vi "6. References.vi"() -> ()   [LabVIEW 2017]
uses:
  6276dcbc-c98b-42be-a14e-8777d527878b.vi
  f718c417-406b-4765-8f4e-f4eec60edb5e.vi
  6276dcbc-c98b-42be-a14e-8777d527878b.vi/b09b9099-6be0-413b-8afc-4908471460c3.vi
  f718c417-406b-4765-8f4e-f4eec60edb5e.vi/b09b9099-6be0-413b-8afc-4908471460c3.vi
  INI-Static-Variable-Support/_Support/global-csm-ini-db-change-flag.vi
  <vilib>/Utility/Data Type/Get Type Information.vi
  <userlib>/_NEVSTOP/Communicable State Machine(CSM)/addons/API-String-Arugments-Support/_Support/Data To SingleElementsArray_csm.vi
  INI-Static-Variable-Support/_Support/Parse Used Session and Name.vi
  <userlib>/_NEVSTOP/Communicable State Machine(CSM)/addons/API-String-Arugments-Support/_Support/Data To API String Arguments.vi
  INI-Static-Variable-Support/_Support/INI-FGV.vi
  <userlib>/_NEVSTOP/Communicable State Machine(CSM)/addons/API-String-Arugments-Support/_Support/Convert API String Arguments to Data(variant).vi
  <userlib>/_NEVSTOP/Communicable State Machine(CSM)/addons/API-String-Arugments-Support/_Support/SingleElementsArray To Data_csm.vi
  INI-Static-Variable-Support/INI-Static-Variable-Support.lvlib
panel:
  out "${NETWORK.URL}":string
  out "${RT.ADDR}":string
  out "case1.addr":string
  out "case2.addr":string
  out "config out 2":cluster{"select":string, "addr":string}
  out "${rt.addr}":string
  out "${network.url} 2":string
  out "${network.url}":string
  out "config out":cluster{"url":string, "host":string}
  out "url":string
  out "host":string
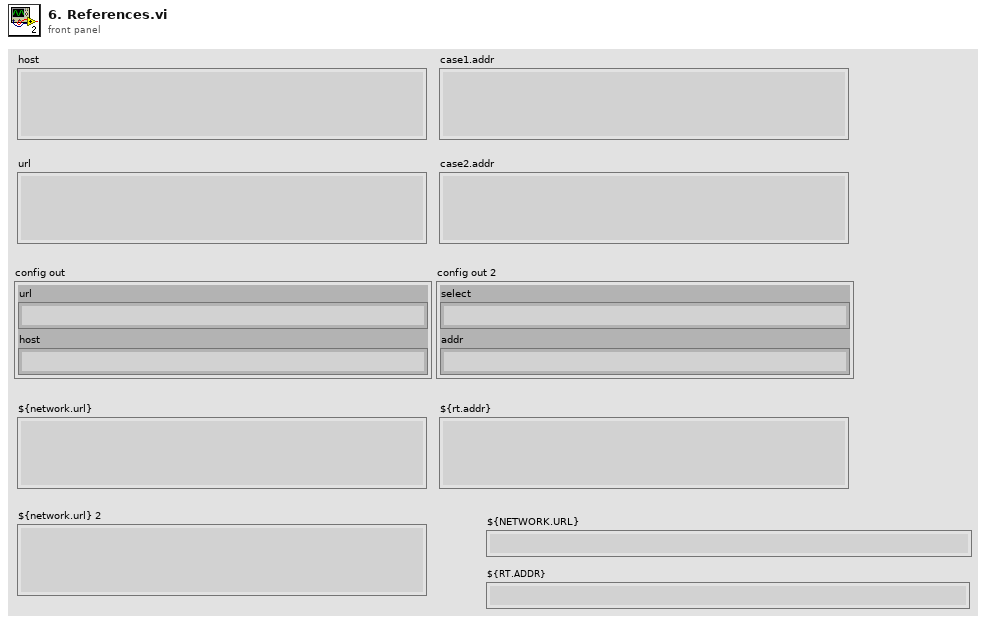
[diagram p1: front panel]
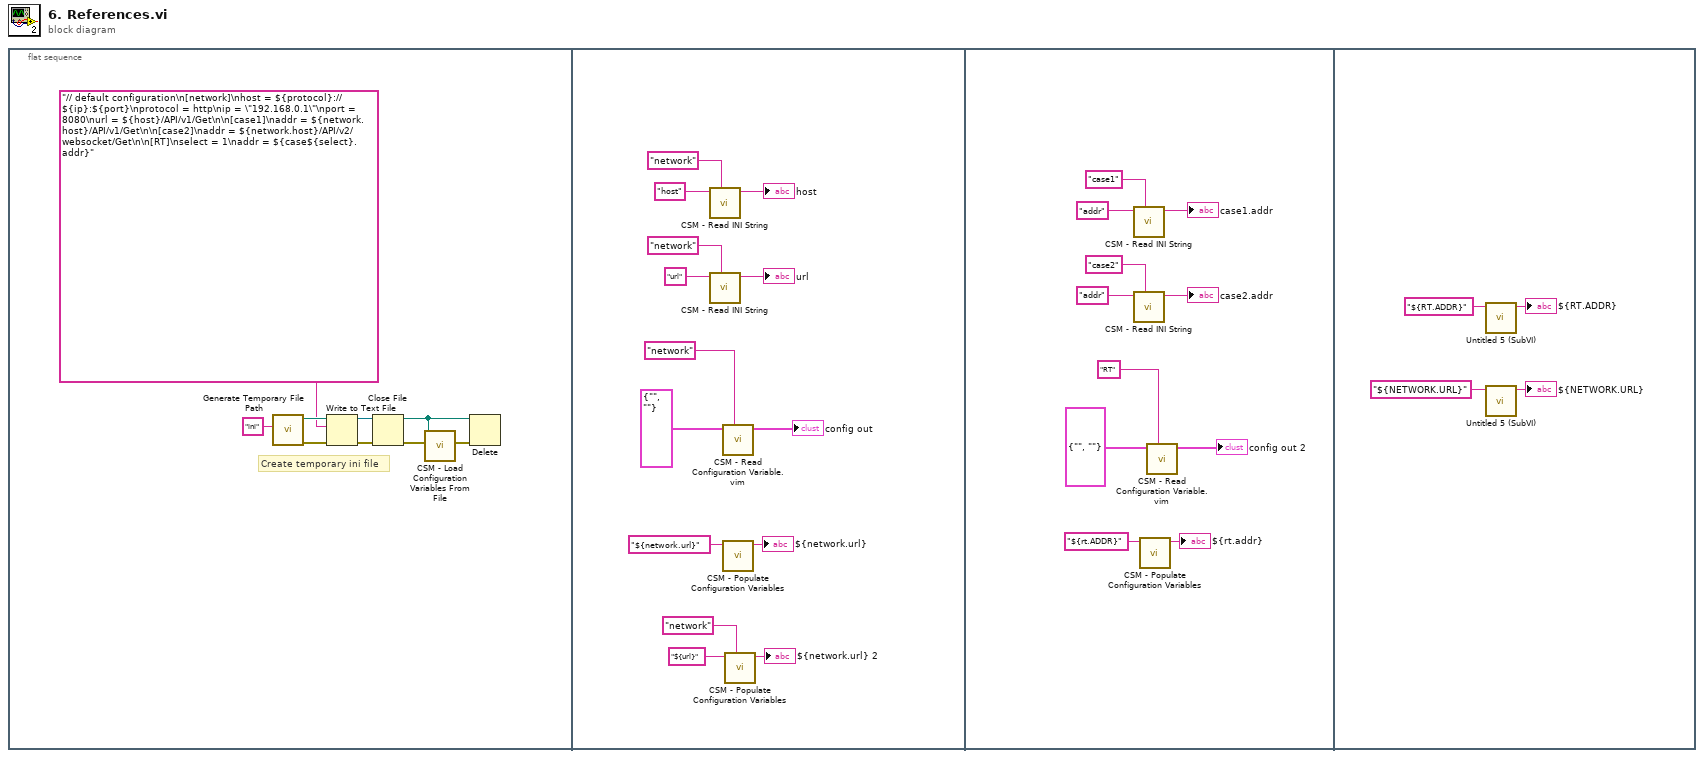
[diagram p0: block diagram]
diagram:
  n1 = flat-sequence {
    frame #0 {
      # "Create temporary ini file"
      n2 = call <vilib>:"Generate Temporary File Path.vi"("Temporary File Extension (tmp)"="ini") -> ("error out"=w9:errorcluster, "Unique Temporary File Path"=w6:path)  [unwired: 9 in]
      n3 = Write to Text File(file (use dialog)=w6, text="// default configuration\n[network]\nhost = ${protocol}://${ip}:${port}\nprotocol = http\nip = \"192.168.0.1\"\nport = 8080\nurl = ${host}/API/v1/Get\n\n[case1]\naddr = ${network.host}/API/v1/Get\n\n[case2]\naddr = ${network.host}/API/v2/websocket/Get\n\n[RT]\nselect = 1\naddr = ${case${select}.addr}", error in=w9) -> (refnum out=w5:refnum<file>, error out=w7:errorcluster)  [unwired: 1 in, 1 out]
      n4 = Close File(refnum=w5, error in=w7) -> (path=w1:path, error out=w4:errorcluster)
      n5 = call "CSM - Load Configuration Variables From File.vi"("error in (no error)"=w4, "Path"=w1) -> ("error out"=w2:errorcluster)  [unwired: 7 in]
      n6 = Delete(path (use dialog)=w1, error in=w2) -> ()  [unwired: 3 in, 3 out]
    }
    frame #1 {
      n7 = call "CSM - Read INI String.vi"("Section Name(\"\" as Default)"="network" ("Section Name(\"\" as Default)"), "String in"="host") -> ("String out"=→"host":string)  [unwired: 5 in, 2 out]
      n8 = call "CSM - Read INI String.vi"("Section Name(\"\" as Default)"="network" ("Section Name(\"\" as Default)"), "String in"="url") -> ("String out"=→"url":string)  [unwired: 5 in, 2 out]
      n9 = call "CSM - Read Configuration Variable.vim"("Section Name(\"\" as Default)"="network" ("Section Name(\"\" as Default)"), "config prototype(Cluster Prefered)"=cluster{"url":string, "host":string} {"url"="", "host"=""}) -> ("config out"=→"config out":cluster{"url":string, "host":string})  [unwired: 6 in, 1 out]
      n10 = call "CSM - Populate Configuration Variables.vi"("String in"="${network.url}") -> ("String out"=→"${network.url}":string)  [unwired: 7 in, 1 out]
      n11 = call "CSM - Populate Configuration Variables.vi"("Section Name(\"\" as Default)"="network" ("Section Name(\"\" as Default)"), "String in"="${url}") -> ("String out"=→"${network.url} 2":string)  [unwired: 6 in, 1 out]
    }
    frame #2 {
      n12 = call "CSM - Read INI String.vi"("Section Name(\"\" as Default)"="case1" ("Section Name(\"\" as Default)"), "String in"="addr") -> ("String out"=→"case1.addr":string)  [unwired: 5 in, 2 out]
      n13 = call "CSM - Read INI String.vi"("Section Name(\"\" as Default)"="case2" ("Section Name(\"\" as Default)"), "String in"="addr") -> ("String out"=→"case2.addr":string)  [unwired: 5 in, 2 out]
      n14 = call "CSM - Populate Configuration Variables.vi"("String in"="${rt.ADDR}") -> ("String out"=→"${rt.addr}":string)  [unwired: 7 in, 1 out]
      n15 = call "CSM - Read Configuration Variable.vim"("Section Name(\"\" as Default)"="RT" ("Section Name(\"\" as Default)"), "config prototype(Cluster Prefered)"=cluster{"select":string, "addr":string} {"select"="", "addr"=""}) -> ("config out"=→"config out 2":cluster{"select":string, "addr":string})  [unwired: 6 in, 1 out]
    }
    frame #3 {
      n16 = call "Untitled 5 (SubVI).vi"("String might with variables"="${RT.ADDR}" ("String in 3")) -> ("String out"=→"${RT.ADDR}":string)  [unwired: 9 in, 1 out]
      n17 = call "Untitled 5 (SubVI).vi"("String might with variables"="${NETWORK.URL}" ("String in 3")) -> ("String out"=→"${NETWORK.URL}":string)  [unwired: 9 in, 1 out]
    }
  }
